vi "XIPIN_LMB_BRAM_Controller_4_0.vi"   [LabVIEW 2017]
doc: "Local Memory Bus (LMB) Block RAM (BRAM) Interface Controller connects to an lmb bus\n------------------------------------\n<b>Need License</b> : No\n<b>Interface</b> : AXI4"
uses:
  <vilib>/rvi/XilinxIP/XIPIN_XNode/niFpgaXIPIN.xnode
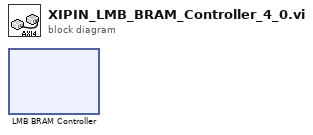
[diagram p0: block diagram]
diagram:
  n1 = xnode ("LMB BRAM Controller")() -> ()
